vi "BattLoad.vi"() -> ()   [LabVIEW 2025]
uses:
  Config.ctl
  Range.ctl
  Mode.ctl
  State.ctl
  Globals.vi
  <vilib>/Instr/_visa.llb/VISA Configure Serial Port (Instr).vi
panel:
  out "Rtemp":dbl caption="Resistor's temp(C)" format="%#_5g"
  in  "Graph":bool caption="Config"
  in  "File":path
  in  "PathBtn":path
  out "SetVisible":bool
  in  "Start":bool
  out "Init":bool
  in  "exit":bool
  in  "Connect":bool
  in  "TabCtrl":enum32{"Graph", "Config"}(tab)
  out "Wh":dbl format="%#_4g"
  out "Chart":cluster{dbl[], dbl[]}[](graph)
  out "Ah":dbl format="%#_4f"
  out "V":dbl format="%#_5g"
  out "A":dbl format="%#_4g"
  in  "SaveCfgPico":bool
  in  "Config":T1={"Pico"="COM5", "Range"=enum."0.26", "Mode"=enum."Serial", "R"=[0.19948381185531616, 0.39327406883239746, 0.3932740092277527]}
  out "Msg":string
  in  "Calibrate":bool
  in  "CalCur":sgl=5.0 caption="Cal Current"
  # "R1 Only"
  # "Parallel"
  # "Serial"
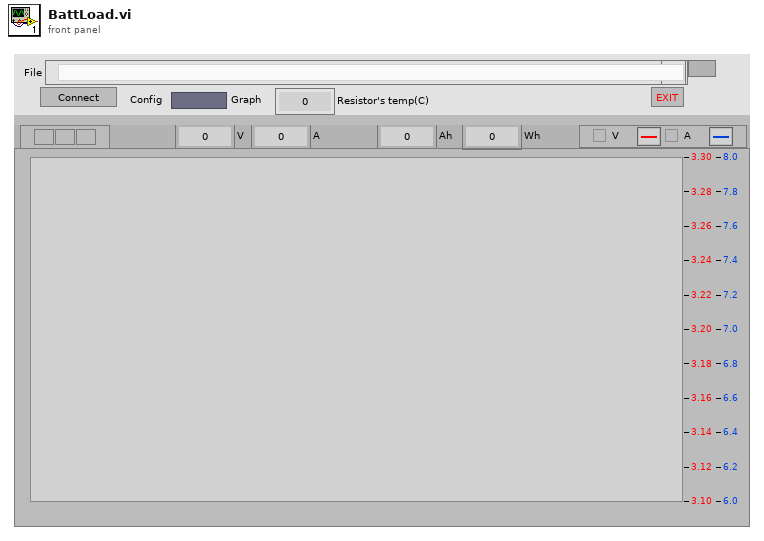
[diagram p1: front panel]
types:
  T1 = typedef "Config.ctl" = cluster{"Pico":refnum<visa-resource-name>, "Range":T2, "Mode":T3, "R":dbl[]}
  T2 = typedef "Range.ctl" = enum16{"0.26", "0.52", "1.03", "2.05", "4.1", "6.2"}
  T3 = typedef "Mode.ctl" = enum16{"R1 Only", "Parallel", "Serial"}
  T4 = typedef "State.ctl" = enum16{"Idle", "Connected", "Calibrating", "Running", "Sync"}
  T5 = enum16{"Left Button", "Center Button", "Right Button", "Window Close"}
  T6 = enum16{"open", "replace", "create", "open or create", "replace or create", "replace or create with confirmation"}
  T7 = enum8{"Enabled", "Disabled", "Disabled and Grayed Out"}
  T8 = enum32{"invalid app kind", "Development System", "Run Time System", "Student Edition", "Embedded LabVIEW", "Evaluation", "Custom"}
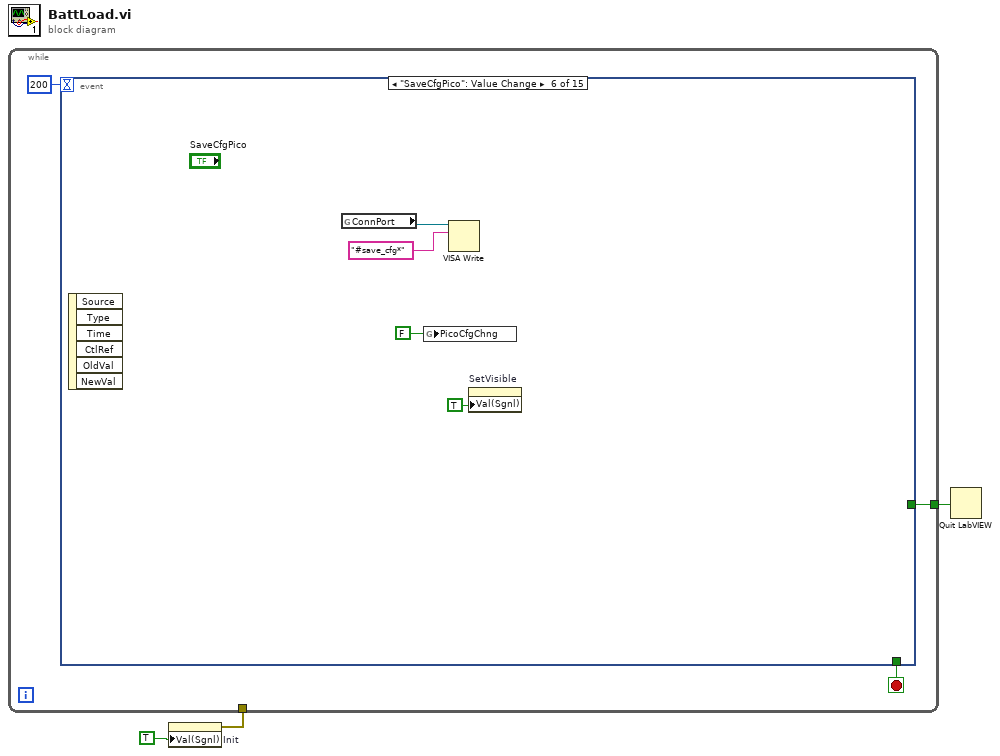
[diagram p0: block diagram]
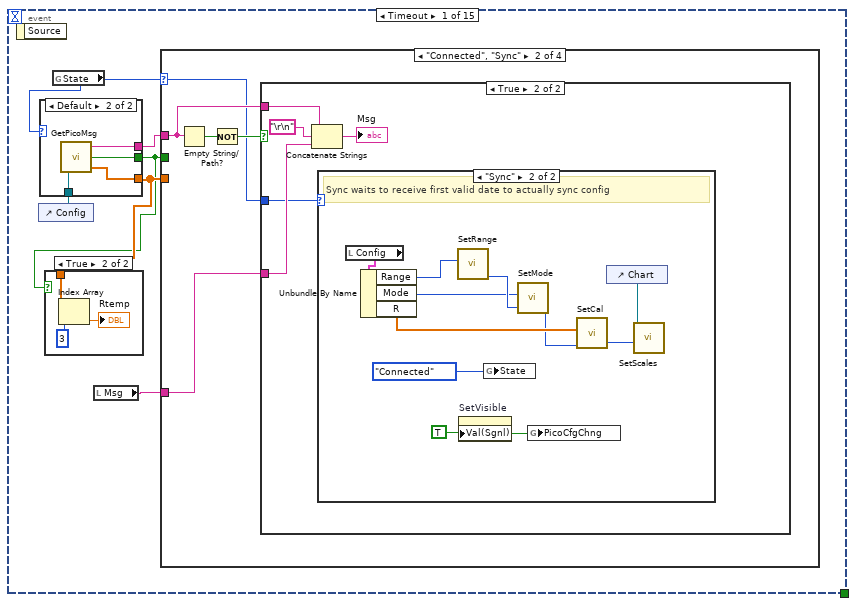
[diagram p2: hidden frame]
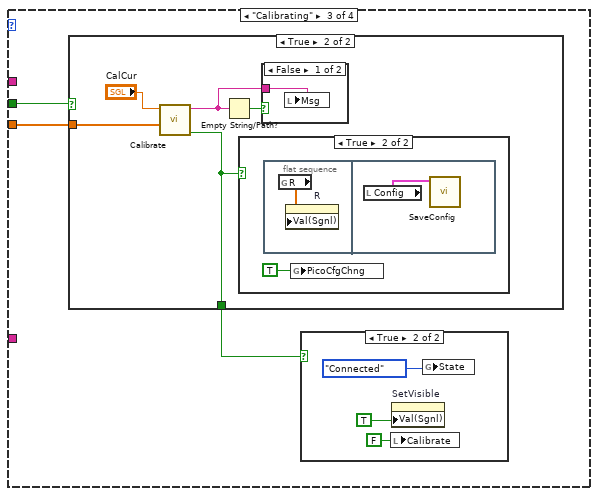
[diagram p8: hidden frame]
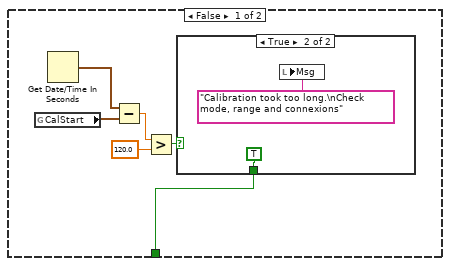
[diagram p10: hidden frame]
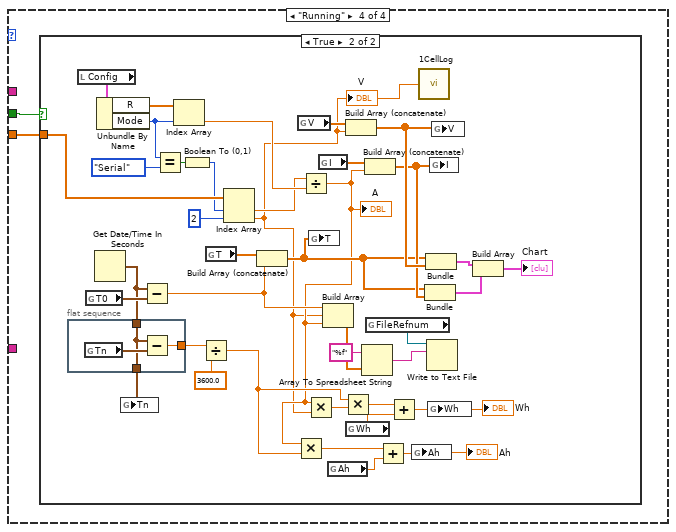
[diagram p14: hidden frame]
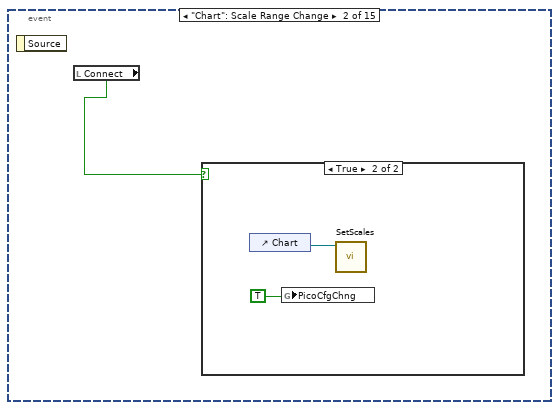
[diagram p16: hidden frame]
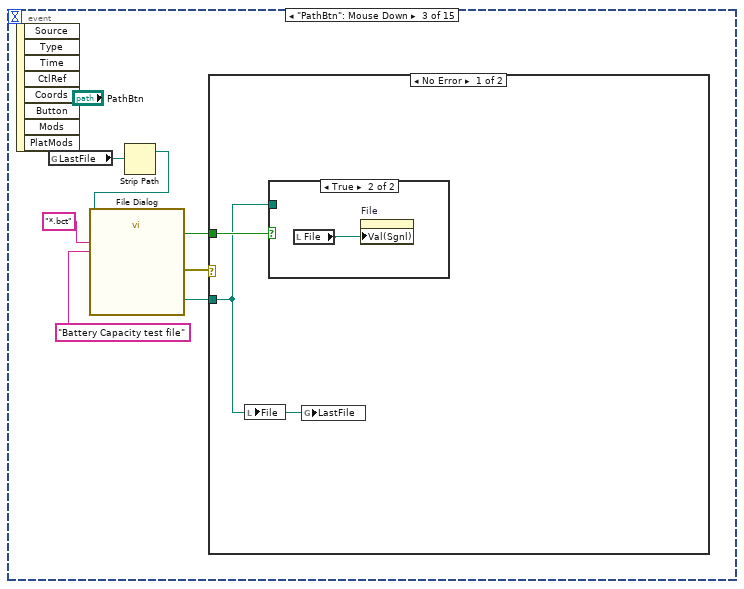
[diagram p18: hidden frame]
diagram:
  n1 = property on="Init" class="Bool (strict)"("Val(Sgnl)"=TRUE) -> (error out=w2:errorcluster)  [unwired: 2 in, 1 out]
  n2 = while {
    tunnel: w2 -> [_]
    tunnel: [w4] -> w1
    stop <- w5 stop-if-true
    n3 = event shown="[5] \"SaveCfgPico\": Value Change" {
      selector: _ -> [_ _ _ _ _ _ _ _ _ _ _ _ _ _ _]
      dyn-events: _ -> [_ _ _ _ _ _ _ _ _ _ _ _ _ _ _]
      timeout: 200 -> [_ _ _ _ _ _ _ _ _ _ _ _ _ _ _]
      tunnel: [_ _ _ _ _ _ _ _ _ _ _ _ "exit" _ _] -> w5
      tunnel: [_ _ _ _ _ _ _ _ _ _ _ _ w274 _ _] -> w4
      event Timeout {
        n4 = event-data() -> ()  [unwired: 1 in, 1 out]
        n5 = control-ref of="Config"() -> (w7:refnum<vi>)
        n6 = global read "Globals.vi" "State"() -> (w12:T4)
        n7 = case shown="Default" w12 {
          tunnel: [_ w19] -> w11
          tunnel: [_ w18] -> w8
          tunnel: [_ w17] -> w9
          tunnel: w7 -> [_ w16]
          frame "Idle" {
          }
          frame Default {
            n8 = call "GetPicoMsg.vi"("CfgRef"=w16) -> ("Values"=w17:dbl[], "Data"=w18:bool, "Msg"=w19:string)  [unwired: 2 in]
          }
        }
        n9 = case shown="True" w8 {
          tunnel: w9 -> [_ w15]
          frame False {
          }
          frame True {
            n10 = Index Array(array=w15, index=3) -> (element=→"Rtemp":dbl)
          }
        }
        n11 = local read "Msg"() -> (w10:string)
        n12 = case shown="\"Connected\", \"Sync\"" w12 {
          selector: w12 -> [_ w20 _ _]
          tunnel: w11 -> [_ w22 _ _]
          tunnel: w8 -> [_ _ w42 w64]
          tunnel: w9 -> [_ _ w41 w63]
          tunnel: w10 -> [_ w21 _ _]
          frame "Idle", Default {
          }
          frame "Connected", "Sync" {
            n13 = Empty String/Path?(string/path=w22) -> (empty?=w24:bool)
            n14 = Not(x=w24) -> (.not. x?=w23:bool)
            n15 = case shown="True" w23 {
              tunnel: w22 -> [_ w27]
              tunnel: w21 -> [_ w26]
              tunnel: w20 -> [_ w25]
              frame False {
              }
              frame True {
                n16 = Concatenate Strings(w27, "\r\n", w26) -> (→"Msg":string)
                n17 = case shown="\"Sync\"" w25 {
                  frame Default {
                  }
                  frame "Sync" {
                    w32 = TRUE
                    # "Sync waits to receive first valid date to actually sync config"
                    n18 = local read "Config"() -> (w39:T1)
                    n19 = Unbundle By Name(w39) -> ("Range"=w38:T2, "Mode"=w36:T3, "R"=w35:dbl[])
                    n20 = call "SetRange.vi"("Range"=w38) -> ("Sleep"=w37:u32)  [unwired: 10 in]
                    n21 = property on="SetVisible" class="Bool (strict)"("Val(Sgnl)"=w32) -> ()  [unwired: 2 in, 2 out]
                    n22 = global write "Globals.vi" "State"(State."Connected" ("State")) -> ()
                    n23 = call "SetMode.vi"("Sleep"=w37, "Mode"=w36) -> ("Sleep"=w34:u32)  [unwired: 9 in]
                    n24 = global write "Globals.vi" "PicoCfgChng"(w32) -> ()
                    n25 = call "SetCal.vi"("Sleep"=w34, "R"=w35) -> ("Sleep"=w31:u32)  [unwired: 9 in]
                    n26 = control-ref of="Chart"() -> (w30:refnum<vi>)
                    n27 = call "SetScales.vi"("Sleep"=w31, "XYGraph in"=w30) -> ()  [unwired: 9 in, 1 out]
                  }
                }
              }
            }
          }
          frame "Calibrating" {
            n28 = case shown="True" w42 {
              tunnel: w41 -> [_ w57]
              tunnel: [w46 w54] -> w40
              frame False {
                n29 = global read "Globals.vi" "CalStart"() -> (w51:timestamp)
                n30 = Get Date/Time In Seconds() -> (seconds since 1Jan1904=w50:timestamp)
                n31 = Subtract(x=w50, y=w51) -> (x-y=w49:dbl)
                n32 = Greater?(x=w49, y=120.0) -> (0:w47:bool)
                n33 = case shown="True" w47 {
                  tunnel: [_ TRUE] -> w46
                  frame False {
                  }
                  frame True {
                    n34 = local write "Msg"("Calibration took too long.\nCheck mode, range and connexions" ("Msg")) -> ()
                  }
                }
              }
              frame True {
                n35 = call "Calibrate.vi"("Voltages"=w57, "CalCurrent"="CalCur") -> ("Done"=w54:bool, "ProgressMsg"=w56:string)  [unwired: 8 in]
                n36 = Empty String/Path?(string/path=w56) -> (empty?=w55:bool)
                n37 = case shown="True" w54 {
                  frame False {
                  }
                  frame True {
                    n38 = flat-sequence {
                      frame #0 {
                        n39 = global read "Globals.vi" "R"() -> (w60:dbl[])
                        n40 = property on="R" class="Arr (strict)"("Val(Sgnl)"=w60) -> ()  [unwired: 2 in, 2 out]
                      }
                      frame #1 {
                        n41 = local read "Config"() -> (w61:T1)
                        n42 = call "SaveConfig.vi"("Config"=w61) -> ()  [unwired: 11 in]
                      }
                    }
                    n43 = global write "Globals.vi" "PicoCfgChng"(TRUE) -> ()
                  }
                }
                n44 = case shown="False" w55 {
                  tunnel: w56 -> [w62 _]
                  frame False {
                    n45 = local write "Msg"(w62) -> ()
                  }
                  frame True {
                  }
                }
              }
            }
            n46 = case shown="True" w40 {
              frame False {
              }
              frame True {
                n47 = local write "Calibrate"(FALSE ("Calibrate")) -> ()
                n48 = property on="SetVisible" class="Bool (strict)"("Val(Sgnl)"=TRUE) -> ()  [unwired: 2 in, 2 out]
                n49 = global write "Globals.vi" "State"(State."Connected" ("State")) -> ()
              }
            }
          }
          frame "Running" {
            n50 = case shown="True" w64 {
              tunnel: w63 -> [_ w101]
              frame False {
              }
              frame True {
                n51 = flat-sequence {
                  tunnel: w79 -> [w105]
                  tunnel: [w105] -> w77
                  tunnel: [w104] -> w76
                  frame #0 {
                    n52 = global read "Globals.vi" "Tn"() -> (w106:timestamp)
                    n53 = Subtract(x=w105, y=w106) -> (x-y=w104:dbl)
                  }
                }
                n54 = local read "Config"() -> (w103:T1)
                n55 = global read "Globals.vi" "T0"() -> (w95:timestamp)
                n56 = Get Date/Time In Seconds() -> (seconds since 1Jan1904=w79:timestamp)
                n57 = Unbundle By Name(w103) -> ("R"=w102:dbl[], "Mode"=w100:T3)
                n58 = global write "Globals.vi" "Tn"(w77) -> ()
                n59 = Subtract(x=w79, y=w95) -> (x-y=w84:dbl)
                n60 = Equal?(x=w100, y=Mode."Serial") -> (x = y?=w98:bool)
                n61 = Index Array(array=w102, index=w100) -> (element=w96:dbl)
                n62 = Boolean To (0,1)(Boolean=w98) -> (0, 1=w97:i16)
                n63 = Divide(x=w76, y=3600.0) -> (x/y=w71:dbl)
                n64 = global read "Globals.vi" "T"() -> (w93:dbl[])
                n65 = Index Array(array=w101, index #1=w97, index #2=2 ("index")) -> (element #1=w91:dbl, element #2=w65:dbl)
                "V" <- w65
                n66 = Build Array (concatenate)(w93, w84) -> (w78:dbl[])
                n67 = global read "Globals.vi" "V"() -> (w92:dbl[])
                n68 = Divide(x=w91, y=w96) -> (x/y=w66:dbl)
                "A" <- w66
                n69 = Multiply(x=w66, y=w71) -> (x*y=w69:dbl)
                n70 = Multiply(x=w66, y=w65) -> (x*y=w72:dbl)
                n71 = global write "Globals.vi" "T"(w78) -> ()
                n72 = global read "Globals.vi" "I"() -> (w90:dbl[])
                n73 = Build Array(w84, w65, w66) -> (w83:dbl[])
                n74 = global read "Globals.vi" "Ah"() -> (w70:dbl)
                n75 = Multiply(x=w71, y=w72) -> (x*y=w74:dbl)
                n76 = Build Array (concatenate)(w92, w65) -> (w89:dbl[])
                n77 = global read "Globals.vi" "Wh"() -> (w73:dbl)
                n78 = Array To Spreadsheet String(array=w83, 3:"%f" ("format string")) -> (spreadsheet string=w80:string)  [unwired: 1 in]
                n79 = Build Array (concatenate)(w90, w66) -> (w88:dbl[])
                n80 = global read "Globals.vi" "FileRefnum"() -> (w81:refnum<file>)
                n81 = Add(x=w69, y=w70) -> (x+y=w68:dbl)
                "Ah" <- w68
                n82 = Add(x=w74, y=w73) -> (x+y=w67:dbl)
                "Wh" <- w67
                n83 = global write "Globals.vi" "Ah"(w68) -> ()
                n84 = call "1CellLog.vi"("CellV"=w65) -> ()  [unwired: 1 in]
                n85 = Bundle(w78, w88) -> (w86:cluster{dbl[], dbl[]})  [unwired: 1 in]
                n86 = Bundle(w78, w89) -> (w87:cluster{dbl[], dbl[]})  [unwired: 1 in]
                n87 = Write to Text File(file (use dialog)=w81, text=w80) -> ()  [unwired: 2 in, 3 out]
                n88 = global write "Globals.vi" "Wh"(w67) -> ()
                n89 = global write "Globals.vi" "I"(w88) -> ()
                n90 = global write "Globals.vi" "V"(w89) -> ()
                n91 = Build Array(w87, w86) -> (→"Chart":cluster{dbl[], dbl[]}[])
              }
            }
          }
        }
      }
      event "Chart": Scale Range Change {
        n92 = event-data() -> ()  [unwired: 1 in, 1 out]
        n93 = local read "Connect"() -> (w107:bool)
        n94 = case shown="True" w107 {
          frame False {
          }
          frame True {
            n95 = control-ref of="Chart"() -> (w108:refnum<vi>)
            n96 = global write "Globals.vi" "PicoCfgChng"(TRUE) -> ()
            n97 = call "SetScales.vi"("XYGraph in"=w108) -> ()  [unwired: 10 in, 1 out]
          }
        }
      }
      event "PathBtn": Mouse Down {
        n98 = event-data() -> ()  [unwired: 1 in, 8 out]
        n99 = global read "Globals.vi" "LastFile"() -> (w111:path)
        n100 = Strip Path(path=w111) -> (stripped path=w110:path)  [unwired: 1 out]
        n101 = call "File Dialog"("start path"=w110, "pattern (all files)"="*.bct", "pattern label"="Battery Capacity test file") -> ("selected path"=w113:path, "exists"=w112:bool, "error out"=w114:errorcluster)  [unwired: 9 in, 1 out]
        n102 = case shown="No Error" w114 {
          tunnel: w113 -> [w117 _]
          tunnel: w112 -> [w118 _]
          frame No Error {
            n103 = local write "File"(w117) -> ()
            n104 = case shown="True" w118 {
              tunnel: w117 -> [_ _]
              frame False {
              }
              frame True {
                n105 = local read "File"() -> (w119:path)
                n106 = property on="File" class="Path"("Val(Sgnl)"=w119) -> ()  [unwired: 2 in, 2 out]
              }
            }
            n107 = global write "Globals.vi" "LastFile"(w117) -> ()
          }
          frame Error {
          }
        }
      }
      event "Start": Value Change {
        n108 = event-data() -> ()  [unwired: 1 in, 1 out]
        n109 = case shown="False" "Start" {
          frame False {
            n110 = global read "Globals.vi" "FileRefnum"() -> (w123:refnum<file>)
            n111 = global write "Globals.vi" "State"(State."Connected" ("State")) -> ()
            n112 = Close File(refnum=w123) -> ()  [unwired: 1 in, 2 out]
          }
          frame True {
            w125 = State."Running" ("State")
            n113 = Empty String/Path?(string/path="File") -> (empty?=w144:bool)
            n114 = case shown="True" w144 {
              tunnel: [w181 w184] -> w132
              tunnel: "File" -> [w181 _]
              frame False {
              }
              frame True {
                n115 = global read "Globals.vi" "LastFile"() -> (w182:path)
                n116 = Strip Path(path=w182) -> (stripped path=w183:path)  [unwired: 1 out]
                n117 = Build Path(base path=w183, name or relative path="TestFile.bct") -> (appended path=w184:path)
                n118 = local write "File"(w184) -> ()
              }
            }
            n119 = call <vilib>:"Check if File or Folder Exists.vi"("path"=w132) -> ("file or folder exists?"=w131:bool)  [unwired: 8 in, 2 out]
            n120 = case shown="False" w131 {
              tunnel: [T5."Left Button" ("Which Button?") w176] -> w133
              frame False {
              }
              frame True {
                w177 = "File exists" ("message")
                n121 = call <vilib>:"Three Button Dialog.vi"("Allow user to close window? (TRUE)"=FALSE, "Window Title (\"\")"=w177, "Center Button Text (\"No\")"="Append" ("Left Button Text (\"Yes\")"), "Left Button Text (\"Yes\")"="Overwrite" ("Left Button Text (\"Yes\")"), "message"=w177) -> ("Which Button?"=w176:T5)  [unwired: 6 in]
              }
            }
            n122 = case shown="Default" w133 {
              tunnel: [w155 w158] -> w138
              tunnel: [_ w162] -> w142
              tunnel: [_ w161] -> w141
              tunnel: [_ w160] -> w140
              tunnel: w132 -> [_ w159]
              tunnel: [_ w157] -> w139
              tunnel: [w155 w156] -> w137
              tunnel: [TRUE _] -> w135
              frame Default {
                w154 = 0.0 ("Ah")
                n123 = Get Date/Time In Seconds() -> (seconds since 1Jan1904=w155:timestamp)
                n124 = global write "Globals.vi" "Wh"(w154) -> ()
                n125 = global write "Globals.vi" "Ah"(w154) -> ()
              }
              frame "Center Button" {
                n126 = call "LoadData.vi"("File"=w159) -> ("Rel_T0"=w158:timestamp, "I"=w160:dbl[], "V"=w161:dbl[], "T"=w162:dbl[], "Chart"=w157:cluster{dbl[], dbl[]}[], "Tn"=w156:timestamp)  [unwired: 5 in]
              }
            }
            n127 = global read "Globals.vi" "State"() -> (w134:T4)
            n128 = global write "Globals.vi" "V"(w141) -> ()
            n129 = global write "Globals.vi" "T"(w142) -> ()
            n130 = global write "Globals.vi" "Tn"(w137) -> ()
            n131 = global write "Globals.vi" "I"(w140) -> ()
            n132 = local write "Chart"(w139) -> ()
            n133 = global write "Globals.vi" "T0"(w138) -> ()
            n134 = case shown="Default" w133 {
              selector: w133 -> [w146 w152]
              tunnel: w132 -> [w149 _]
              tunnel: w131 -> [w148 _]
              tunnel: [w146 w152] -> w130
              tunnel: [w147 _] -> w129
              frame Default {
                n135 = case shown="True" w148 {
                  tunnel: w149 -> [_ w151]
                  tunnel: [_ w150] -> w147
                  frame False {
                  }
                  frame True {
                    n136 = call "BackupFile.vi"("path in"=w151) -> ("error out"=w150:errorcluster)  [unwired: 9 in, 1 out]
                  }
                }
              }
              frame "Right Button" {
              }
            }
            n137 = Select(t=T5."Right Button" ("Which Button?"), s=w129, f=w130) -> (s? t:f=w127:T5)
            n138 = case shown="\"Center Button\"" w127 {
              tunnel: w132 -> [w164 w171 _]
              tunnel: w125 -> [w163 w173 _]
              tunnel: [w163 w173 w174] -> w126
              tunnel: [w166 w168 _] -> w143
              tunnel: w135 -> [_ _ _]
              tunnel: w134 -> [_ _ w174]
              frame "Left Button" {
                # "Overwrite"
                # "Overwrite Existing"
                n139 = Open/Create/Replace File(file path (use dialog)=w164, operation (0:open)=T6."replace or create") -> (refnum out=w166:refnum<file>)  [unwired: 4 in, 2 out]
              }
              frame "Center Button" {
                # "Append"
                # "Append"
                n140 = Open/Create/Replace File(file path (use dialog)=w171, operation (0:open)=T6."open") -> (refnum out=w169:refnum<file>, error out=w170:errorcluster)  [unwired: 4 in, 1 out]
                n141 = Set File Position(refnum=w169, from (0:start)=enum16{"start", "end", "current"}."end", error in=w170) -> (refnum out=w168:refnum<file>)  [unwired: 1 in, 1 out]
              }
              frame Default {
                # "Cancel"
              }
            }
            n142 = global write "Globals.vi" "FileRefnum"(w143) -> ()
            n143 = Equal?(x=w125, y=w126) -> (x = y?=w124:bool)
            n144 = global write "Globals.vi" "State"(w126) -> ()
            n145 = case shown="True" w124 {
              selector: w124 -> [_ w145]
              frame False {
              }
              frame True {
                n146 = property on="Graph" class="Bool (strict)"("Val(Sgnl)"=w145) -> ()  [unwired: 2 in, 2 out]
              }
            }
          }
        }
        n147 = property on="SetVisible" class="Bool (strict)"("Val(Sgnl)"=TRUE) -> ()  [unwired: 2 in, 2 out]
      }
      event Value Change {
        n148 = event-data() -> ("OldVal"=w203:T1, "NewVal"=w195:T1)  [unwired: 1 in]
        n149 = call "SaveConfig.vi"("Config"=w195) -> ()  [unwired: 11 in]
        n150 = Unbundle By Name(w195) -> ("Range"=w193:T2, "Mode"=w186:T3, "R"=w200:dbl[])
        n151 = Unbundle By Name(w203) -> ("Range"=w202:T2, "Mode"=w187:T3, "R"=w201:dbl[])
        n152 = local read "Connect"() -> (w196:bool)
        n153 = Not Equal?(x=w201, y=w200) -> (x != y?=w199:bool)
        n154 = Not Equal?(x=w202, y=w193) -> (x != y?=w198:bool)
        n155 = And(x=w196, y=w199) -> (x .and. y?=w194:bool)
        n156 = Not Equal?(x=w186, y=w187) -> (x != y?=w191:bool)
        n157 = And(x=w196, y=w198) -> (x .and. y?=w192:bool)
        n158 = Compound Arithmetic op=OR(w191, w198, w199) -> (w197:bool)
        n159 = call "SetRange.vi"("DoIt"=w192, "Range"=w193) -> ("Sleep"=w190:u32)  [unwired: 9 in]
        n160 = case shown="True" w197 {
          frame False {
          }
          frame True {
            n161 = local write "Msg"("") -> ()
            n162 = global write "Globals.vi" "PicoCfgChng"(TRUE) -> ()
          }
        }
        n163 = And(x=w196, y=w191) -> (x .and. y?=w188:bool)
        n164 = call "SetMode.vi"("Sleep"=w190, "DoIt"=w188, "Mode"=w186) -> ("Sleep"=w189:u32)  [unwired: 8 in]
        n165 = call "SetCal.vi"("Sleep"=w189, "DoIt"=w194, "R"=w200) -> ()  [unwired: 8 in, 1 out]
      }
      event "SaveCfgPico": Value Change {
        n166 = event-data() -> ()  [unwired: 1 in, 6 out]
        n167 = global read "Globals.vi" "ConnPort"() -> (w209:refnum<visa-resource-name>)
        n168 = global write "Globals.vi" "PicoCfgChng"(FALSE) -> ()
        n169 = VISA Write(VISA resource name=w209, write buffer="#save_cfg*") -> ()  [unwired: 1 in, 3 out]
        n170 = property on="SetVisible" class="Bool (strict)"("Val(Sgnl)"=TRUE) -> ()  [unwired: 2 in, 2 out]
      }
      event "Graph": Value Change {
        n171 = event-data() -> ()  [unwired: 1 in, 6 out]
        n172 = Select(t=enum32{"Graph", "Config"}."Graph" ("TabCtrl"), s="Graph", f=enum32{"Graph", "Config"}."Config" ("TabCtrl")) -> (s? t:f=w210:enum32{"Graph", "Config"})
        n173 = local write "TabCtrl"(w210) -> ()
      }
      event "File": Mouse Down {
        n174 = event-data() -> ("Mods.Double Click"=w214:bool)  [unwired: 1 in]
        n175 = case shown="True" w214 {
          frame False {
          }
          frame True {
            n176 = local read "File"() -> (w215:path)
            n177 = property on="File" class="Path"("Val(Sgnl)"=w215) -> ()  [unwired: 2 in, 2 out]
          }
        }
      }
      event "File": Value Change {
        n178 = event-data() -> ("NewVal"=w217:path)  [unwired: 1 in, 5 out]
        n179 = flat-sequence {
          tunnel: w217 -> [w219]
          frame #0 {
            n180 = call "LoadData.vi"("File"=w219) -> ("Chart"=w218:cluster{dbl[], dbl[]}[])  [unwired: 5 in, 5 out]
            n181 = local write "Chart"(w218) -> ()
          }
          frame #1 {
            n182 = global read "Globals.vi" "Wh"() -> (w220:dbl)
            n183 = global read "Globals.vi" "Ah"() -> (w221:dbl)
            n184 = local write "Ah"(w221) -> ()
            n185 = local write "Wh"(w220) -> ()
          }
        }
        n186 = property on="Graph" class="Bool (strict)"("Val(Sgnl)"=TRUE) -> ()  [unwired: 2 in, 2 out]
      }
      event "Msg": Mouse Down {
        n187 = event-data() -> ("Mods.Double Click"=w222:bool)  [unwired: 1 in]
        n188 = case shown="True" w222 {
          frame False {
          }
          frame True {
            n189 = local write "Msg"("") -> ()
          }
        }
      }
      event "Calibrate": Value Change {
        n190 = event-data() -> ()  [unwired: 1 in, 6 out]
        n191 = case shown="True" "Calibrate" {
          tunnel: [State."Connected" ("State") State."Calibrating" ("State")] -> w225
          frame False {
          }
          frame True {
            n192 = Get Date/Time In Seconds() -> (seconds since 1Jan1904=w231:timestamp)
            n193 = global write "Globals.vi" "Calibration"(sgl[] [] ("Calibration")) -> ()
            n194 = property on="Msg" class="Str"("Visible"=TRUE ("Blinking"), "Value"="Calibration started" ("Msg")) -> ()  [unwired: 2 in, 2 out]
            n195 = global write "Globals.vi" "CalStart"(w231) -> ()
          }
        }
        n196 = global write "Globals.vi" "State"(w225) -> ()
        n197 = property on="SetVisible" class="Bool (strict)"("Val(Sgnl)"=TRUE ("Value (Signaling)")) -> ()  [unwired: 2 in, 2 out]
      }
      event "Connect": Value Change {
        n198 = event-data() -> ()  [unwired: 1 in, 1 out]
        n199 = property on="Pico" class="VISAName"() -> ("Value"=w236:refnum<visa-resource-name>)  [unwired: 2 in, 2 out]
        n200 = case shown="True" "Connect" {
          tunnel: w236 -> [_ w266]
          tunnel: [w259 w264] -> w235
          tunnel: State."Idle" ("State") -> [w259 w263]
          tunnel: [_ w262] -> w233
          frame False {
            n201 = global read "Globals.vi" "ConnPort"() -> (w261:refnum<visa-resource-name>)
            n202 = VISA Close(VISA resource name=w261) -> (error out=w260:errorcluster)  [unwired: 1 in]
            n203 = call <vilib>:"Clear Errors.vi"("error in (no error)"=w260) -> ()  [unwired: 5 in, 2 out]
          }
          frame True {
            n204 = call-poly "VISA Configure Serial Port"("VISA resource name"=w266) -> ("VISA resource name out"=w262:refnum<visa-resource-name>, "error out"=w265:errorcluster)  [unwired: 13 in]
            n205 = case shown="No Error" w265 {
              tunnel: w262 -> [w267 _]
              tunnel: [State."Sync" ("State") w272] -> w264
              tunnel: w263 -> [_ w272]
              frame No Error {
                n206 = global write "Globals.vi" "ConnPort"(w267) -> ()
                n207 = property on="Range" class="Enum (strict)"() -> ("Value"=w268:T2)  [unwired: 2 in, 2 out]
                n208 = property on="Msg" class="Str"("Visible"=TRUE, "Value"="") -> ()  [unwired: 2 in, 2 out]
                n209 = property on="Range" class="Enum (strict)"("Val(Sgnl)"=w268) -> ()  [unwired: 2 in, 2 out]
              }
              frame Error {
                n210 = local write "Connect"(FALSE) -> ()
                n211 = call <vilib>:"Beep.vi"() -> ()  [unwired: 12 in]
              }
            }
          }
        }
        n212 = case shown="\"Sync\"" w235 {
          tunnel: [T7."Enabled" ("Disabled") T7."Disabled and Grayed Out" ("Disabled")] -> w234
          tunnel: w233 -> [_ w242]
          frame "Idle", Default {
          }
          frame "Sync" {
            n213 = flat-sequence {
              tunnel: w246 -> [_]
              tunnel: w242 -> [w258]
              tunnel: [w257] -> w244
              tunnel: [w257] -> w241
              frame #0 {
                n214 = property class="Instr"(reference=w258) -> ("Serial Settings:Number of Bytes at Serial Port"=w257:u32)  [unwired: 1 in, 2 out]
              }
            }
            n215 = Wait (ms)(milliseconds to wait=u32 200) -> (millisecond timer value=w246:u32)
            n216 = Equal To 0?(x=w244) -> (x = 0?=w243:bool)
            n217 = case shown="True" w243 {
              tunnel: w242 -> [_ w249]
              tunnel: w241 -> [_ w248]
              frame False {
              }
              frame True {
                n218 = stacked-sequence {
                  tunnel: w249 -> [w251 w254 w256]
                  tunnel: w248 -> [w250 _ _]
                  frame #0 {
                    n219 = VISA Read(VISA resource name=w251, byte count=w250) -> ()  [unwired: 1 in, 4 out]
                  }
                  frame #1 {
                    w253 = "\u0002"  # CTRL b
                    n220 = VISA Write(VISA resource name=w254, write buffer=w253) -> ()  [unwired: 1 in, 3 out]
                    n221 = Wait (ms)(milliseconds to wait=u32 200) -> ()  [unwired: 1 out]
                  }
                  frame #2 {
                    w255 = "\u0004"  # CTRLd
                    n222 = VISA Write(VISA resource name=w256, write buffer=w255) -> ()  [unwired: 1 in, 3 out]
                  }
                }
              }
            }
          }
        }
        n223 = global write "Globals.vi" "State"(w235) -> ()
        n224 = property on="SetVisible" class="Bool (strict)"("Val(Sgnl)"=TRUE) -> ()  [unwired: 2 in, 2 out]
        n225 = property on="Pico" class="VISAName"("DisabledEnum"=w234) -> ()  [unwired: 2 in, 2 out]
      }
      event "exit": Value Change {
        n226 = event-data() -> ()  [unwired: 1 in, 6 out]
        n227 = local read "Connect"() -> (w277:bool)
        n228 = case shown="True" w277 {
          tunnel: [_ w279] -> _
          frame False {
          }
          frame True {
            n229 = global read "Globals.vi" "ConnPort"() -> (w280:refnum<visa-resource-name>)
            n230 = VISA Close(VISA resource name=w280) -> (error out=w279:errorcluster)  [unwired: 1 in]
          }
        }
        n231 = property class="App"() -> ("App.Kind"=w276:T8)  [unwired: 2 in, 2 out]
        n232 = Equal?(x=w276, y=T8."Run Time System") -> (x = y?=w274:bool)
      }
      event "Init": Value Change {
        w282 = FALSE
        n233 = event-data() -> ()  [unwired: 1 in, 6 out]
        n234 = flat-sequence {
          frame #0 {
            # "Default"
            n235 = call <vilib>:"Application Directory.vi"() -> ("Application Directory"=w287:path)
            n236 = Build Path(base path=w287, name or relative path=path "Data") -> (appended path=w286:path)
            n237 = Build Path(base path=w286, name or relative path=path "Tst1.bct") -> (appended path=w289:path)
            n238 = global write "Globals.vi" "LastFile"(w289) -> ()
            n239 = call <vilib>:"Check if File or Folder Exists.vi"("path"=w286) -> ("file or folder exists?"=w292:bool, "dup path"=w291:path)  [unwired: 8 in, 1 out]
            n240 = case shown="False" w292 {
              tunnel: w291 -> [w293 _]
              frame False {
                n241 = Create Folder(path (use dialog)=w293) -> ()  [unwired: 2 in, 3 out]
              }
              frame True {
              }
            }
          }
          frame #1 {
            n242 = call "LoadConfig.vi"() -> ("Config"=w294:T1)  [unwired: 11 in]
            n243 = local write "Config"(w294) -> ()
          }
        }
        n244 = property on="Chart" class="XYGraph (strict)"("Value"=cluster{dbl[], dbl[]}[] [] ("Chart")) -> ()  [unwired: 2 in, 2 out]
        n245 = local write "Graph"(w282) -> ()
        n246 = local write "Connect"(w282) -> ()
        n247 = property on="Msg" class="Str"("Visible"=w282) -> ()  [unwired: 2 in, 2 out]
        n248 = local write "Start"(w282) -> ()
        n249 = property on="SetVisible" class="Bool (strict)"("Val(Sgnl)"=TRUE) -> ()  [unwired: 2 in, 2 out]
        n250 = global write "Globals.vi" "State"(State."Idle" ("State")) -> ()
        n251 = local write "TabCtrl"(enum32{"Graph", "Config"}."Config" ("TabCtrl")) -> ()
        "Init" <- w282
      }
      event "SetVisible": Value Change {
        w299 = T7."Disabled and Grayed Out" ("Disabled")
        w300 = T7."Enabled" ("Disabled")
        n252 = event-data() -> ()  [unwired: 1 in, 6 out]
        n253 = global read "Globals.vi" "State"() -> (w311:T4)
        n254 = local read "Connect"() -> (w297:bool)
        n255 = Equal?(x=State."Calibrating", y=w311) -> (x = y?=w307:bool)
        n256 = local read "Start"() -> (w306:bool)
        n257 = Not(x=w307) -> (.not. x?=w309:bool)
        n258 = property on="Calibrate" class="Bool (strict)"("Blinking"=w307) -> ()  [unwired: 2 in, 2 out]
        n259 = Not(x=w306) -> (.not. x?=w305:bool)
        n260 = And(x=w297, y=w305) -> (x .and. y?=w308:bool)
        n261 = And(x=w309, y=w297) -> (x .and. y?=w312:bool)
        n262 = Or(x=w307, y=w306) -> (x .or. y?=w303:bool)
        n263 = property on="Start" class="Bool (strict)"("Visible"=w312) -> ()  [unwired: 2 in, 2 out]
        n264 = Select(t=w300, s=w308, f=w299) -> (s? t:f=w301:T7)
        n265 = Select(t=w299, s=w303, f=w300) -> (s? t:f=w302:T7)
        n266 = Select(t=w300, s=w305, f=w299) -> (s? t:f=w304:T7)
        n267 = global read "Globals.vi" "PicoCfgChng"() -> (w295:bool)
        n268 = property on="Range" class="Enum (strict)"("DisabledEnum"=w302) -> ()  [unwired: 2 in, 2 out]
        n269 = And(x=w297, y=w295) -> (x .and. y?=w296:bool)
        n270 = property on="Config" class="Clust (strict)"("DisabledEnum"=w304) -> ()  [unwired: 2 in, 2 out]
        n271 = Select(t=w300, s=w296, f=w299) -> (s? t:f=w298:T7)
        n272 = property on="Calibrate" class="Bool (strict)"("DisabledEnum"=w301) -> ()  [unwired: 2 in, 2 out]
        n273 = property on="CalCur" class="DigNum (strict)"("DisabledEnum"=w301) -> ()  [unwired: 2 in, 2 out]
        n274 = property on="SaveCfgPico" class="Bool"("DisabledEnum"=w298) -> ()  [unwired: 2 in, 2 out]
        n275 = property on="Connect" class="Bool (strict)"("DisabledEnum"=w304) -> ()  [unwired: 2 in, 2 out]
        n276 = property on="exit" class="Bool"("DisabledEnum"=w304) -> ()  [unwired: 2 in, 2 out]
        "SetVisible" <- FALSE ("SetVisible")
      }
    }
  }
  n277 = Quit LabVIEW(quit? (T)=w1) -> ()
